vi "Cmd Get Parameters.vi"(4 "error in (no error)":errorcluster, 6 "ADODB.Parameters":refnum<k7>) -> (0 "error out":errorcluster, 2 "ADODB.Parameters out":refnum<k7>, 3 "parameters":T1[](array[typedef]))   [LabVIEW 2020, in "NI_Database_API.lvlib"]
doc: "Returns an array of parameter information associated with the ADODB.Parameters refnum."
uses:
  <vilib>/addons/database/NI_Database_API.lvlib
  <vilib>/addons/database/Auxilliary.llb/DB Tools Parameter Info.ctl
  <vilib>/addons/database/Auxilliary.llb/DB Tools DataTypes.ctl
  <vilib>/addons/database/Auxilliary.llb/DB Tools Parameter Dir.ctl
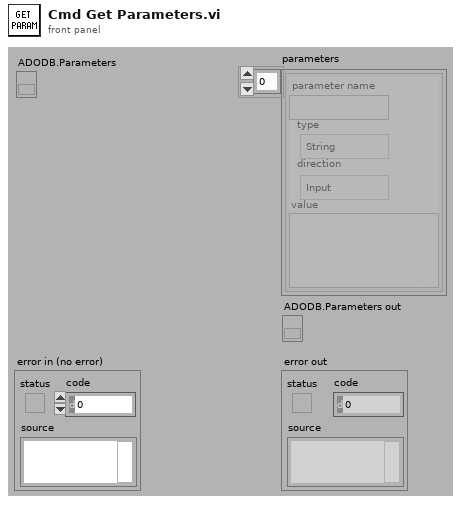
[diagram p1: front panel]
types:
  T1 = typedef "NI_Database_API.lvlib/DB Tools Parameter Info.ctl" = cluster{"parameter name":string, "type":T2, "direction":T3, "value":variant}
  T2 = typedef "NI_Database_API.lvlib/DB Tools DataTypes.ctl" = enum16{"String", "Long (I32)", "Single (SGL)", "Double (DBL)", "Date/Time", "Binary"}
  T3 = typedef "NI_Database_API.lvlib/DB Tools Parameter Dir.ctl" = enum32{"Input", "Output", "Input/Output", "Return Value"}
  T4 = cluster{"Name":string, "data type":T2, "direction":T3, "Value":variant}
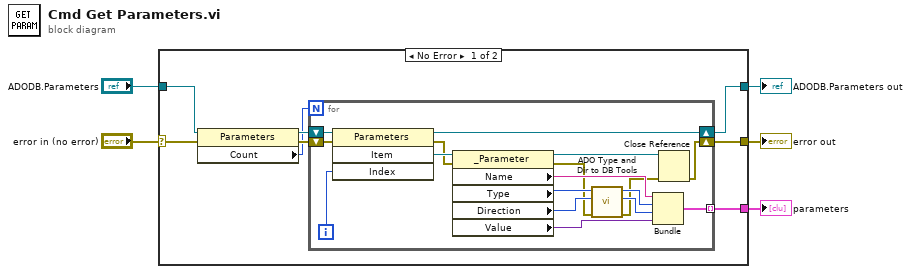
[diagram p0: block diagram]
diagram:
  n1 = case shown="No Error" "error in (no error)" {
    selector: "error in (no error)" -> [w6 w32]
    tunnel: "ADODB.Parameters" -> [w10 w31]
    tunnel: [w9 w31] -> w4
    tunnel: [w8 w32] -> w3
    tunnel: [w7 _] -> w2
    frame No Error {
      n2 = property class="Parameters"(reference=w10, error in=w6) -> (reference out=w12:refnum<k7>, error out=w13:errorcluster, "Count"=w11:i32)
      n3 = for {
        N: w11 -> [_]
        shift-right: [w22] -> w8
        shift-left: w13 -> [w23]
        tunnel: [w21] -> w7 mode=indexing
        shift-right: [w17] -> w9
        shift-left: w12 -> [w30]
        i -> [w29]
        n4 = invoke class="Parameters" method="Item"(reference=w30, error in=w23, "Index"=w29) -> (reference out=w17:refnum<k7>, error out=w27:errorcluster, "Item"=w28:refnum<k7>)  [unwired: 1 in, 1 out]
        n5 = property class="_Parameter"(reference=w28, error in=w27) -> (reference out=w24:refnum<k7>, error out=w16:errorcluster, "Name"=w26:string, "Type"=w20:i32, "Direction"=w19:i32, "Value"=w25:variant)
        n6 = call <vilib>:"ADO Type and Dir to DB Tools.vi"("error in (no error)"=w16, "ADO direction"=w19, "ADO type"=w20) -> ("error out"=w14:errorcluster, "direction"=w15:T3, "data type"=w18:T2)  [unwired: 2 in]
        n7 = Bundle("Name"=w26, "data type"=w18, "direction"=w15, "Value"=w25) -> (w21:T4)  [unwired: 1 in]
        n8 = Close Reference(reference=w24, error in (no error)=w14) -> (error out=w22:errorcluster)
      }
    }
    frame Error {
    }
  }
  "error out" <- w3
  "ADODB.Parameters out" <- w4
  "parameters" <- w2
